vi "DELETEsetLogMode.vi"(8 "error in (no error)":errorcluster, 11 "Instrument.Lockin in":refnum<class "Instrument.Lockin.lvclass">) -> (0 "error out":errorcluster, 3 "Instrument.Lockin out":refnum<class "Instrument.Lockin.lvclass">)   [LabVIEW 2019]
doc: "Set the state {start, stop, reset, start sweep, stop sweep}"
uses:
  Instrument.Lockin/Instrument.Lockin.lvclass
  Instrument.Lockin/Typedefs/API/Lockin.Commands--Enum.ctl
  Instrument.Lockin/Typedefs/API/Lockin.setLogMode--cluster.ctl
panel:
  in  "Interval (s)":dbl
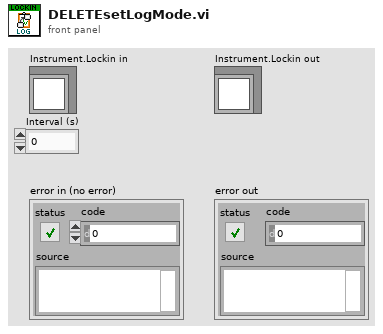
[diagram p1: front panel]
types:
  T1 = typedef "Instrument.Lockin.lvlib/Instrument.Lockin.lvclass/Lockin.setLogMode--cluster.ctl" = cluster{"interval":u32}
  T2 = typedef "Instrument.Lockin.lvlib/Instrument.Lockin.lvclass/Lockin.Commands--Enum.ctl" = enum16{"setAO", "setAO_Amplitude", "setAO_DC", "setAO_Frequency", "setAO_Phase", "setAO_Function", "setREF", "setREF_Frequency", "setREF_Phase", "setREF_TC", "setREF_Roll-Off", "setDAQ", "setSampling", "setState", "getState", "getAO", "getAI", "getResults", "getSampling", "getAOconfig", "getREFconfig", "setInputGain", "setOutputGain", "getInputGain", "getOutputGain", "setSamplingFsMode", "getSamplingFsMode", "setSweep", "setSweep_Time", "setSweep_Table", "getStatus", "getSweepResults", "getSweepWaveforms", "enableLogging", "disableLogging"}
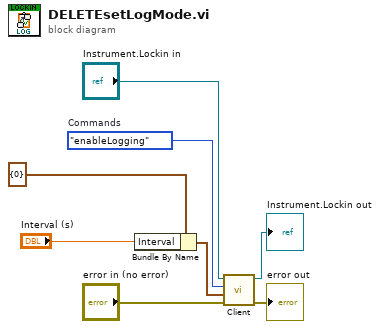
[diagram p0: block diagram]
diagram:
  w6 = Lockin.Commands--Enum."enableLogging"  # Commands
  n1 = Bundle By Name(cluster=T1 {"interval"=0} ("setLogging"), "Interval"="Interval (s)") -> (w7:T1)
  n2 = call-dynamic "Client.vi"("error in (no error)"="error in (no error)", "Data in"=w7, "Command in"=w6, "Instrument in"="Instrument.Lockin in") -> ("error out"=→"error out":errorcluster, "Instrument out"=→"Instrument.Lockin out":refnum<class "Instrument.Lockin.lvclass">)  [unwired: 4 in, 2 out]
